vi "HEWH PRAT Valves.vi"(7 "Normally Closed Valve?":bool, 8 "error in (no error)":errorcluster, 9 "Normally Open Valve":T1, 10 "Station ID":T2=enum."A", 11 "MW100 In":refnum<visa-resource-name>) -> (0 "error out":errorcluster, 2 "Send Command":string, 3 "MW100 Out":refnum<visa-resource-name>)   [LabVIEW 2023]
uses:
  Type Definitions/Station ID Selector.ctl
  Type Definitions/HEWH Normally Open Valve Control.ctl
  Type Definitions/PRAT Channel Settings.ctl
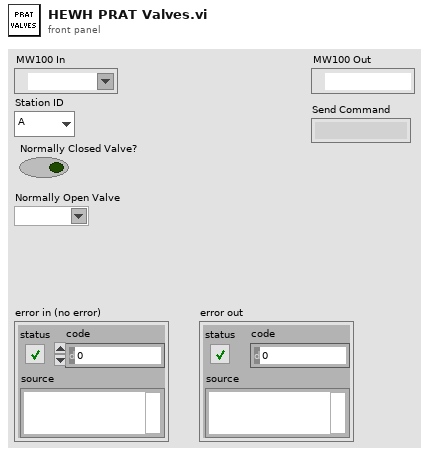
[diagram p1: front panel]
types:
  T1 = typedef "HEWH Normally Open Valve Control.ctl" = string
  T2 = typedef "Station ID Selector.ctl" = enum16{"", "A", "B", "C", "D", "Global"}
  T3 = typedef "LVComboBoxStrsAndValuesArrayTypeDef.ctl" = cluster{"String":string, "Value":string}[]
  T4 = typedef "PRAT Channel Settings.ctl" = string
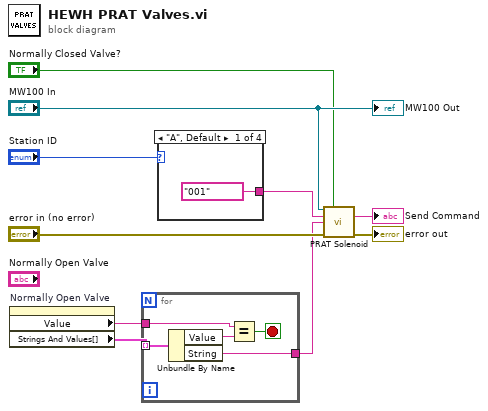
[diagram p0: block diagram]
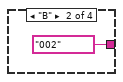
[diagram p2: hidden frame]
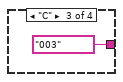
[diagram p3: hidden frame]
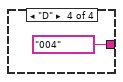
[diagram p4: hidden frame]
diagram:
  n1 = property on="Normally Open Valve" class="CmbBox (strict)"() -> ("Value"=w3:T1, "Strings And Values[]"=w2:T3)  [unwired: 2 in, 2 out]
  n2 = for {
    tunnel: w2 -> [w15] mode=indexing
    tunnel: [w12] -> w1
    tunnel: w3 -> [w11]
    stop <- w13 stop-if-true
    n3 = Unbundle By Name(w15) -> ("Value"=w14:string, "String"=w12:string)
    n4 = Equal?(x=w11, y=w14) -> (x = y?=w13:bool)
  }
  n5 = case shown="\"A\", Default" "Station ID" {
    tunnel: [T4 "001" ("PRAT Channels") T4 "002" ("PRAT Channels") T4 "003" ("PRAT Channels") T4 "004" ("PRAT Channels")] -> w10
    frame "A", Default {
    }
    frame "B" {
    }
    frame "C" {
    }
    frame "D" {
    }
  }
  n6 = call "PRAT Solenoid.vi"("VISA session"="MW100 In", "Normally Closed Valve?"="Normally Closed Valve?", "PRAT Channels"=w10, "Valve Status"=w1, "Error In"="error in (no error)") -> ("Send Command"=→"Send Command":string, "Error Out"=→"error out":errorcluster)  [unwired: 8 in, 1 out]
  "MW100 Out" <- "MW100 In"
